vi "DevTests_CircleVertices.vi"(9 "Center":T2, 10 "Radius":sgl, 11 "Quality":i32) -> (2 "Draw Order":i32[](array[numeric]), 3 "Vertices":T1[](array[typedef]))   [LabVIEW 2026]
uses:
  SDL3/Rect/FPoint--cluster.ctl
  SDL3/Render/Vertex--cluster.ctl
  SDL3/Pixels/FColor--cluster.ctl
  SDL3/Rect/Rect.lvlib
  SDL3/Pixels/Pixels.lvlib
  SDL3/Render/Render.lvlib
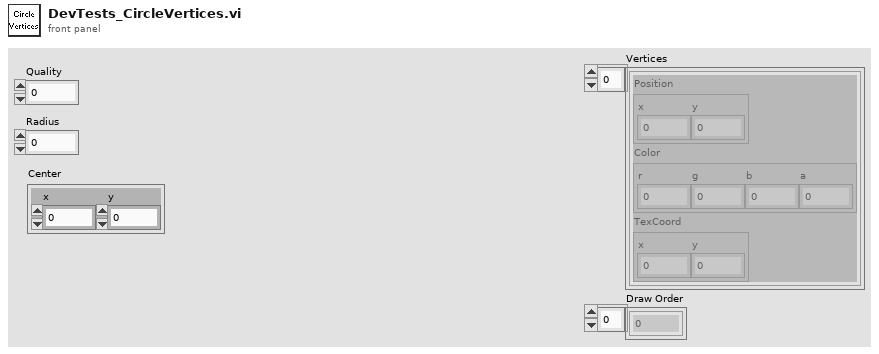
[diagram p1: front panel]
types:
  T1 = typedef "SDL3.lvlib/Render.lvlib/Vertex--cluster.ctl" = cluster{"Position":T2, "Color":T3, "TexCoord":T2}
  T2 = typedef "SDL3.lvlib/Rect.lvlib/FPoint--cluster.ctl" = cluster{"x":sgl, "y":sgl}
  T3 = typedef "SDL3.lvlib/Pixels.lvlib/FColor--cluster.ctl" = cluster{"r":sgl, "g":sgl, "b":sgl, "a":sgl}
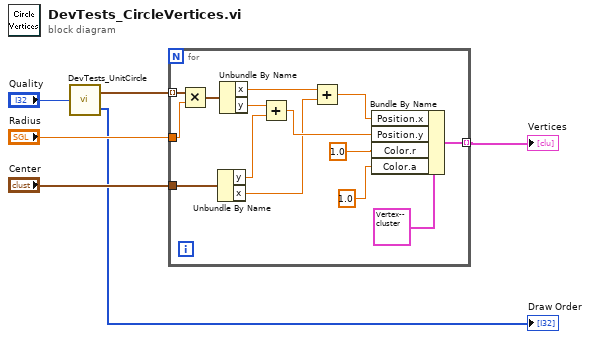
[diagram p0: block diagram]
diagram:
  n1 = call "DevTests_UnitCircle.vi"("Quality"="Quality") -> ("Circle"=w6:T2[], "Order"=→"Draw Order":i32[])
  n2 = for {
    tunnel: w6 -> [w18] mode=indexing
    tunnel: [w19] -> w2 mode=indexing
    tunnel: "Radius" -> [w11]
    tunnel: "Center" -> [w10]
    n3 = Multiply(x=w18, y=w11) -> (x*y=w13:T2)
    n4 = Unbundle By Name(w10) -> ("y"=w9:sgl, "x"=w8:sgl)
    n5 = Unbundle By Name(w13) -> ("x"=w17:sgl, "y"=w16:sgl)
    n6 = Add(x=w16, y=w9) -> (x+y=w14:sgl)
    n7 = Add(x=w17, y=w8) -> (x+y=w15:sgl)
    n8 = Bundle By Name(cluster=T1 {"Position"={"x"=0.0, "y"=0.0}, "Color"={"r"=0.0, "g"=0.0, "b"=0.0, "a"=0.0}, "TexCoord"={"x"=0.0, "y"=0.0}} ("Vertex"), "Position.x"=w15, "Position.y"=w14, "Color.r"=sgl 1.0, "Color.a"=sgl 1.0) -> (w19:T1)
  }
  "Vertices" <- w2
